vi "checkFilesAndSaveHealthcheck.vi"(4 "Disable Automatic Error Handling":bool=TRUE, 6 "Remove Compiled Code":bool=TRUE, 7 "saveBadOnly?":bool, 8 "Resave if changed":bool=TRUE, 9 "filesToCheck":path[](array[path]), 11 "saveTo":path) -> (0 "Broken VIs found":i32, 1 "Progress Bar":i32(slide), 2 "Table":string[][](table))   [LabVIEW 2022 SP3]
uses:
  <vilib>/Utility/error.llb/Trim Whitespace One-Sided.vi
  <vilib>/Utility/file.llb/Write Delimited Spreadsheet (string).vi
panel:
  in  "openBad":bool=TRUE
  out "nFiles":i32
  out "checking":path
  in  "Abort":bool
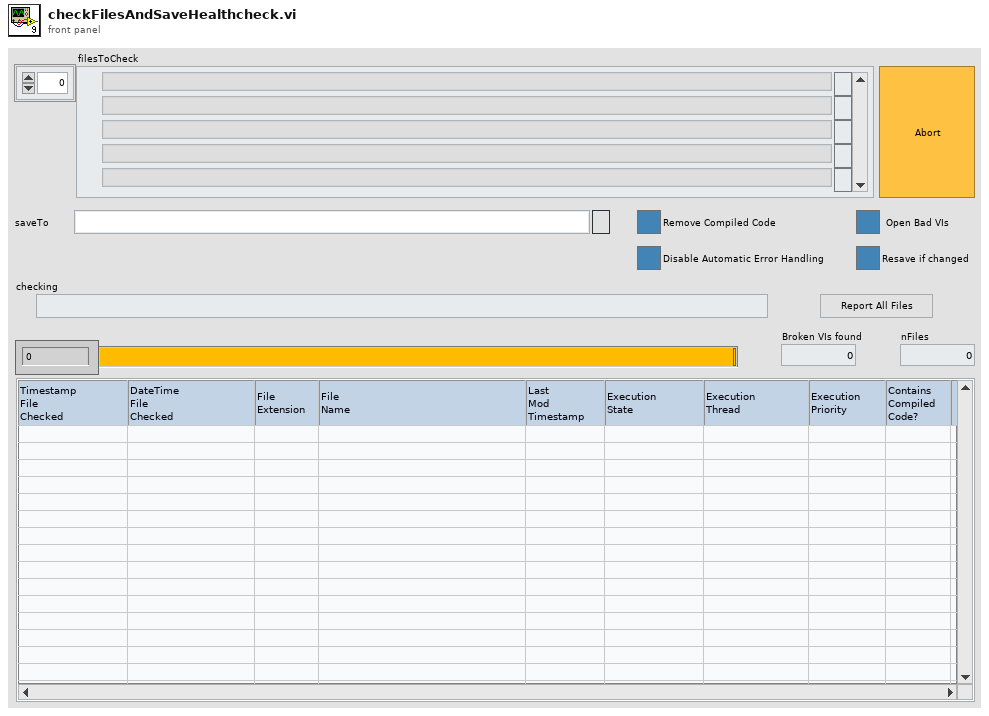
[diagram p1: front panel]
types:
  T1 = typedef "Librarian File Info Out.ctl" = cluster{"creation date":u32, "last mod date":u32, "type":string, "creator":string, "LV version":i32, "size":i32, "top level":bool}
  T2 = enum32{"Bad", "Idle", "Run top level", "Running"}
  T3 = typedef "LVRowAndColumnUnsignedTypeDef.ctl" = cluster{"Row":u32, "Column":u32}
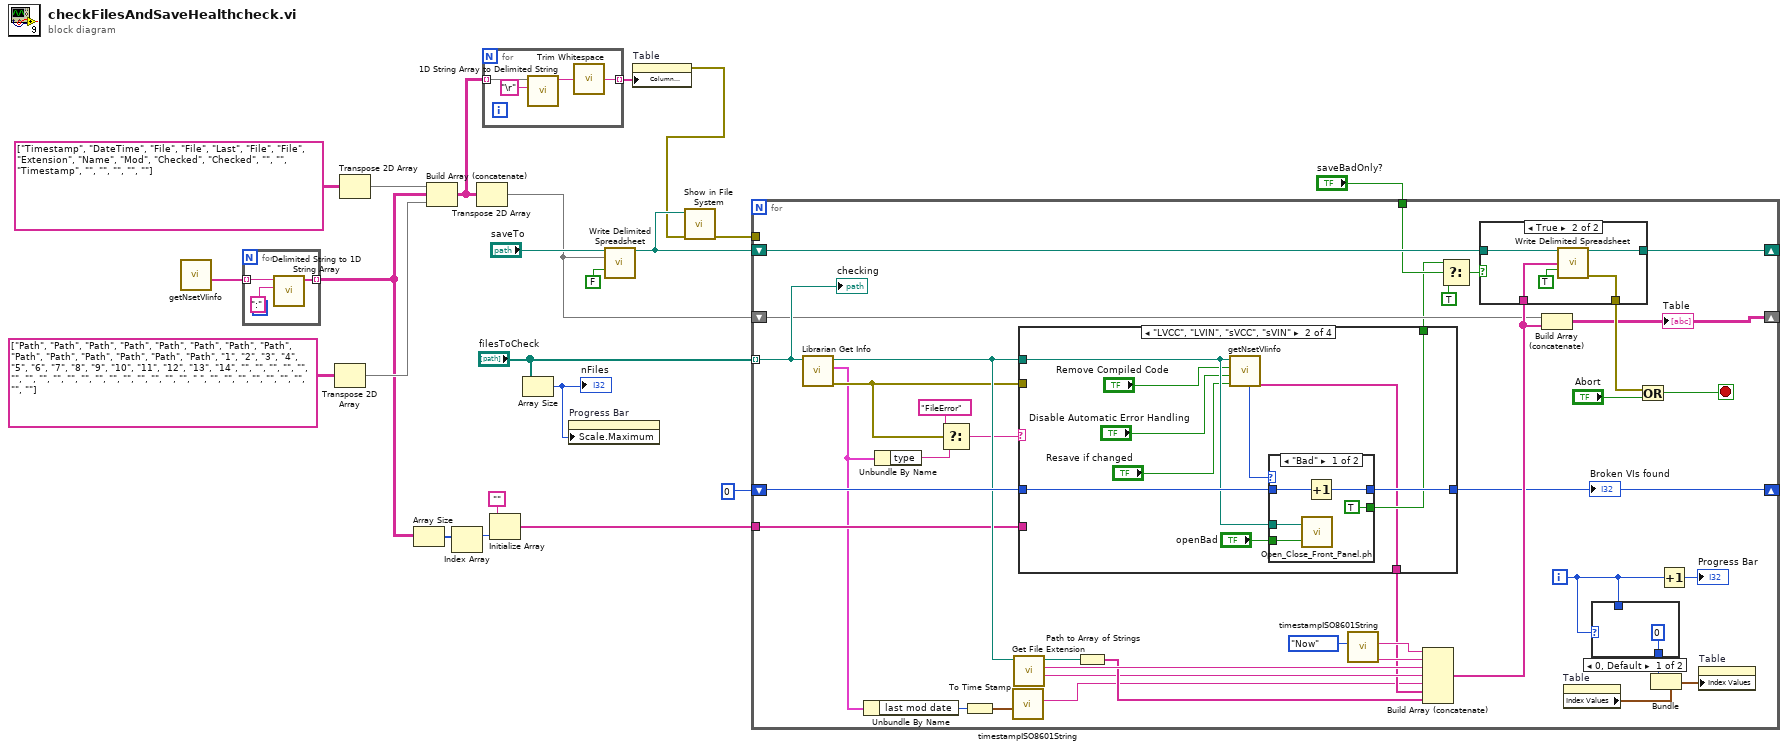
[diagram p0: block diagram]
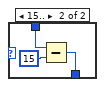
[diagram p2: hidden frame]
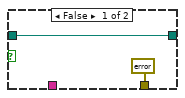
[diagram p3: hidden frame]
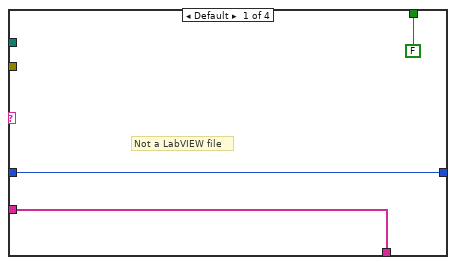
[diagram p4: hidden frame]
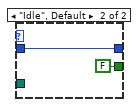
[diagram p5: hidden frame]
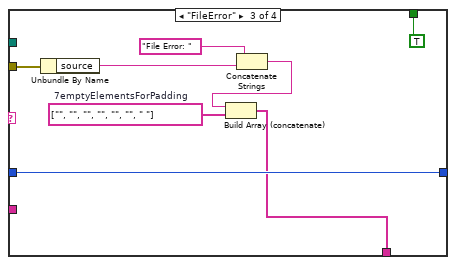
[diagram p6: hidden frame]
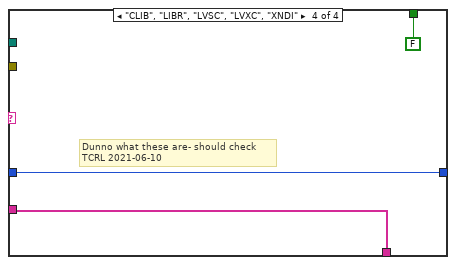
[diagram p7: hidden frame]
diagram:
  n1 = call "getNsetVIinfo.vi"() -> ("titles"=w16:string[])  [unwired: 9 in, 2 out]
  n2 = for {
    tunnel: w16 -> [w24] mode=indexing
    tunnel: [w25] -> w11 mode=indexing
    n3 = call <vilib>:"Delimited String to 1D String Array.vi"("delimiter"=":" ("delimiter (Tab)"), "delimited string"=w24) -> ("string array"=w25:string[])  [unwired: 9 in]
  }
  n4 = Transpose 2D Array(2D array=string[][] [["Path", "Path", "Path", "Path", "Path", "Path", "Path", "Path", "Path", "Path", "Path", "Path", "Path", "Path"], ["1", "2", "3", "4", "5", "6", "7", "8", "9", "10", "11", "12", "13", "14"], ["", "", "", "", "", "", "", "", "", "", "", "", "", ""], ["", "", "", "", " ", "", "", "", "", "", "", "", "", ""]]) -> (transposed array=w12:string[][])
  n5 = Transpose 2D Array(2D array=string[][] [["Timestamp", "DateTime", "File", "File", "Last"], ["File", "File", "Extension", "Name", "Mod"], ["Checked", "Checked", "", "", "Timestamp"], ["", "", "", "", ""]]) -> (transposed array=w15:string[][])
  n6 = Array Size(array=w11) -> (size(s)=w10:i32[])
  n7 = Build Array (concatenate)(w15, w11, w12) -> (w4:string[][])
  n8 = Index Array(array=w10) -> (element=w9:i32)  [unwired: 1 in]
  n9 = Transpose 2D Array(2D array=w4) -> (transposed array=w6:string[][])
  n10 = for {
    tunnel: w4 -> [w29] mode=indexing
    tunnel: [w26] -> w3 mode=indexing
    n11 = call <vilib>:"1D String Array to Delimited String.vi"("delimiter"="\r", "string array"=w29) -> ("delimited string"=w28:string)  [unwired: 9 in]
    n12 = call <vilib>:"Trim Whitespace.vi"("string"=w28) -> ("trimmed string"=w26:string)  [unwired: 1 in]
  }
  n13 = Initialize Array("", w9) -> (w7:string[])
  n14 = Array Size(array="filesToCheck") -> (size(s)=w19:i32)
  "nFiles" <- w19
  n15 = property on="Progress Bar" class="Slide (strict)"("Scale.Maximum"=w19) -> ()  [unwired: 2 in, 2 out]
  n16 = call-poly <vilib>:"Write Delimited Spreadsheet.vi"("file path (dialog if empty)"="saveTo", "2D data"=w6, "append to file? (new file:F)"=FALSE) -> ("new file path (Not A Path if cancelled)"=w5:path)  [unwired: 11 in, 1 out]
  n17 = property on="Table" class="Tbl (strict)"("Column Headers[]"=w3) -> (error out=w2:errorcluster)  [unwired: 2 in, 1 out]
  n18 = call <vilib>:"Show in File System.vi"("error in (no error)"=w2, "file or directory path"=w5) -> ("error out"=w1:errorcluster)  [unwired: 9 in]
  n19 = for {
    tunnel: "filesToCheck" -> [w66] mode=indexing
    shift-right: [w44] -> _
    shift-left: w6 -> [w64]
    shift-right: [w63] -> _
    shift-left: w5 -> [w62]
    shift-right: [w56] -> _
    shift-left: 0 -> [w57]
    tunnel: "saveBadOnly?" -> [w54]
    tunnel: w7 -> [w40]
    tunnel: w1 -> [_]
    i -> [w43]
    stop <- w59 stop-if-true
    n20 = call <vilib>:"Librarian Get Info.vi"("path"=w66) -> ("error out"=w36:errorcluster, "file information"=w31:T1, "dup path"=w50:path)  [unwired: 8 in]
    n21 = Unbundle By Name(w31) -> ("last mod date"=w30:u32)
    n22 = Unbundle By Name(w31) -> ("type"=w39:string)
    n23 = Select(t="FileError", s=w36, f=w39) -> (s? t:f=w38:string)
    n24 = To Time Stamp(1:w30) -> (0:w32:timestamp)
    n25 = call "timestampISO8601String.vi"("Time Stamp"=w32) -> ("timestampString"=w33:string)  [unwired: 7 in, 3 out]
    n26 = call <vilib>:"Get File Extension.vi"("file"=w50) -> ("filename without extension"=w42:string, "lowercase file extension"=w51:string, "dup file"=w49:path)  [unwired: 6 in, 2 out]
    n27 = case shown="\"LVCC\", \"LVIN\", \"sVCC\", \"sVIN\"" w38 {
      tunnel: w50 -> [_ w87 _ _]
      tunnel: w57 -> [w81 w91 w106 w109]
      tunnel: [w81 w90 w106 w109] -> w56
      tunnel: [FALSE w89 TRUE FALSE] -> w53
      tunnel: [w79 w88 w102 w107] -> w41
      tunnel: w40 -> [w79 _ _ w107]
      tunnel: w36 -> [_ _ w103 _]
      frame Default {
        # "Not a LabVIEW file"
      }
      frame "LVCC", "LVIN", "sVCC", "sVIN" {
        n28 = call "getNsetVIinfo.vi"("Resave if required"="Resave if changed", "Disable Automatic Error Handling"="Disable Automatic Error Handling", "Remove Compiled Code"="Remove Compiled Code", "path"=w87) -> ("values"=w88:string[], "Execution:State"=w85:T2)  [unwired: 5 in, 1 out]
        n29 = case shown="\"Bad\"" w85 {
          tunnel: w91 -> [w96 w98]
          tunnel: [w95 w98] -> w90
          tunnel: [TRUE FALSE] -> w89
          tunnel: w87 -> [w93 _]
          tunnel: "openBad" -> [w92 _]
          frame "Bad" {
            n30 = call "Open_Close_Front_Panel.ph.vi"("openWindow (T)"=w92, "VI path"=w93) -> ()  [unwired: 1 in, 1 out]
            n31 = Increment(x=w96) -> (x+1=w95:i32)
          }
          frame "Idle", Default {
          }
        }
      }
      frame "FileError" {
        w104 = string[] ["", "", "", "", "", "", " "]  # 7emptyElementsForPadding
        n32 = Unbundle By Name(w103) -> ("source"=w100:string)
        n33 = Concatenate Strings("File Error: " ("String"), w100) -> (w99:string)
        n34 = Build Array (concatenate)(w99, w104) -> (w102:string[])
      }
      frame "CLIB", "LIBR", "LVSC", "LVXC", "XNDI" {
        # "Dunno what these are- should check\nTCRL 2021-06-10"
      }
    }
    "Broken VIs found" <- w56
    n35 = Path to Array of Strings(0:w49) -> (2:w48:string[])  [unwired: 1 out]
    n36 = call "timestampISO8601String.vi"("When?"=enum16{"Now", "Use Input"}."Now") -> ("date/timeWithSeconds"=w61:string, "timestampString"=w60:string)  [unwired: 7 in, 2 out]
    n37 = Build Array (concatenate)(w60, w61, w51, w42, w33, w41, w48) -> (w65:string[])
    n38 = Select(t=w53, s=w54, f=TRUE) -> (s? t:f=w55:bool)
    n39 = case shown="True" w55 {
      tunnel: w65 -> [_ w78]
      tunnel: [w73 w77] -> w63
      tunnel: w62 -> [w73 w76]
      tunnel: [errorcluster {"status"=FALSE, "code"=0, "source"=""} ("error out") w75] -> w58
      frame False {
      }
      frame True {
        n40 = call-poly <vilib>:"Write Delimited Spreadsheet.vi"("file path (dialog if empty)"=w76, "1D data"=w78, "append to file? (new file:F)"=TRUE) -> ("new file path (Not A Path if cancelled)"=w77:path, "error out"=w75:errorcluster)  [unwired: 11 in]
      }
    }
    n41 = Build Array (concatenate)(w64, w65) -> (w44:string[][])
    "Table" <- w44
    n42 = property on="Table" class="Tbl (strict)"() -> ("Index Values"=w34:T3)  [unwired: 2 in, 2 out]
    n43 = case shown="0, Default" w43 {
      tunnel: w43 -> [_ w71]
      tunnel: [0 w70] -> w46
      frame 0, Default {
      }
      frame 15.. {
        n44 = Subtract(x=w71, y=15) -> (x-y=w70:i32)
      }
    }
    n45 = Or(x=w58, y="Abort") -> (x .or. y?=w59:bool)
    n46 = Bundle(cluster=w34, "Row"=w46) -> (w47:T3)  [unwired: 1 in]
    n47 = Increment(x=w43) -> (x+1=→"Progress Bar":i32)
    n48 = property on="Table" class="Tbl (strict)"("Index Values"=w47) -> ()  [unwired: 2 in, 2 out]
    "checking" <- w66
  }
